vi "GOOP_LVClass_CreateNewWizard_Init.vi"(11 "Wizard":u64) -> (1 "Label":string, 2 "Enable Finish":bool, 3 "Enable Next":bool)   [LabVIEW 2020]
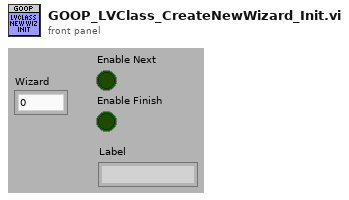
[diagram p1: front panel]
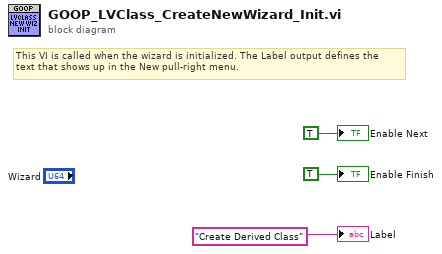
[diagram p0: block diagram]
diagram:
  # "This VI is called when the wizard is initialized. The Label output defines the\ntext that shows up in the New pull-right menu."
  "Enable Next" <- TRUE ("Enable Next")
  "Enable Finish" <- TRUE ("Enable Finish")
  "Label" <- "Create Derived Class" ("Label")
